vi "PH_Sound.set Device Error.vi"(0 "VI in":refnum<vi>, 3 "Device error":errorcluster, 5 "error in":errorcluster) -> (14 "VI out":refnum<vi>, 19 "error out":errorcluster)   [LabVIEW 2014, in "PH_Sound.lvlib"]
uses:
  PH_Sound.lvlib
  PH_Common/PH_Common.lvlib
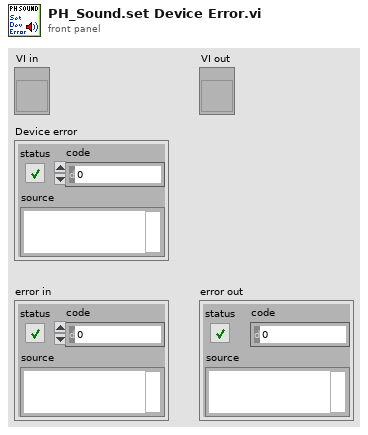
[diagram p1: front panel]
types:
  T1 = typedef "PH_Sound.lvlib/PH_Sound.i attribute.ctl" = cluster{"GUI Refs":cluster{"Exit":refnum<vi>, "Laserfreigabe":refnum<vi>, "PreAmp-Freigabe":refnum<vi>, "Countdown Running":refnum<vi>, "Emergency Off":refnum<vi>, "Device Error":refnum<vi>}, "Testalarm on":bool, "State":cluster{"Laser Class 4":bool, "PreAmp Running":bool, "Countdown Running":bool, "Emergency Off":bool}, "Starting Time":timestamp}
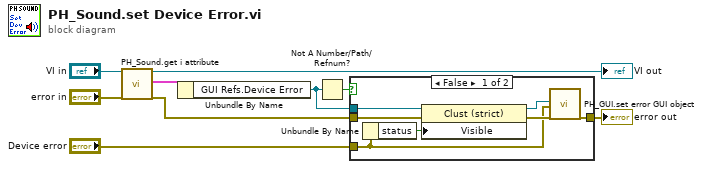
[diagram p0: block diagram]
diagram:
  n1 = call "PH_Sound.get i attribute.vi"("i ref in"="VI in", "error in (no error)"="error in") -> ("i ref out"=→"VI out":refnum<vi>, "i attribute"=w6:T1, "error out"=w4:errorcluster)  [unwired: 15 in]
  n2 = Unbundle By Name(w6) -> ("GUI Refs.Device Error"=w2:refnum<vi>)
  n3 = Not A Number/Path/Refnum?(number/path/refnum=w2) -> (NaN/Path/Refnum?=w3:bool)
  n4 = case shown="False" w3 {
    tunnel: w2 -> [w16 _]
    tunnel: "Device error" -> [w10 _]
    tunnel: w4 -> [w14 w17]
    tunnel: [w12 w17] -> w1
    frame False {
      n5 = Unbundle By Name(w10) -> ("status"=w15:bool)
      n6 = property class="Clust (strict)"(reference=w16, error in=w14, "Visible"=w15) -> (reference out=w11:refnum<vi>, error out=w13:errorcluster)
      n7 = call "PH_GUI.set error GUI object.vi"("GUI Refs.Device Error"=w11, "error to set"=w10, "error in (no error)"=w13) -> ("error out"=w12:errorcluster)  [unwired: 16 in]
    }
    frame True {
    }
  }
  "error out" <- w1
